vi "ConfigureCameraImage.vi"(10 "Image Type":T3 items=["Grayscale (U8)", "Grayscale (I16)", "Grayscale (SGL)", "Complex (CSG)", "RGB (U32)", "HSL (U32)", "RGB (U64)", "Grayscale (U16)"], 11 "Refnum in":T1="cam0") -> (1 "Camera Image":T2, 3 "Refnum out":T1)   [LabVIEW 2013]
doc: "Configure the stuff needed to talk to the camera above the pool for the little boats."
uses:
  <vilib>/userdefined/High Color/IMAQdx.ctl
  <vilib>/vision/Image Controls.llb/IMAQ Image.ctl
  <vilib>/vision/driver/NI_Vision_Acquisition_Software.lvlib
panel:
  out "error out":errorcluster
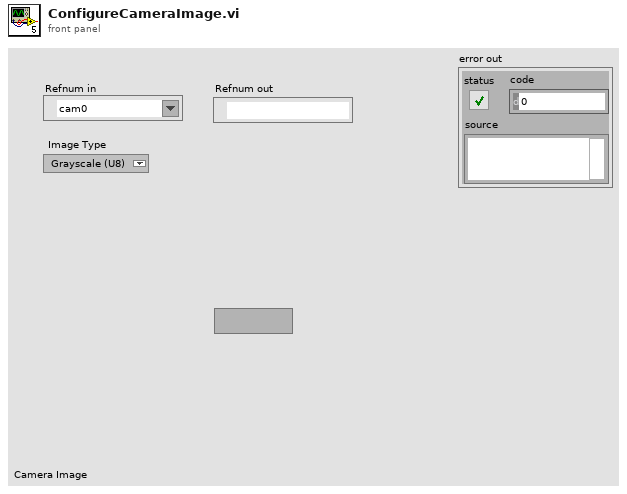
[diagram p1: front panel]
types:
  T1 = typedef "IMAQdx.ctl" = refnum<k21>
  T2 = typedef "IMAQ Image.ctl" = refnum<image>
  T3 = typedef "Image Type" = u32
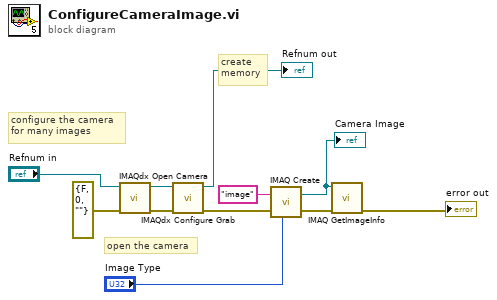
[diagram p0: block diagram]
diagram:
  # "create\nmemory"
  # "configure the camera\nfor many images"
  # "open the camera"
  n1 = call <vilib>:"IMAQdx Open Camera.vi"("error in"=errorcluster {"status"=FALSE, "code"=0, "source"=""}, "Session In"="Refnum in") -> ("error out"=w5:errorcluster, "Session Out"=w4:T1)  [unwired: 1 in, 7 out]
  n2 = call <vilib>:"IMAQdx Configure Grab.vi"("error in"=w5, "Session In"=w4) -> ("error out"=w3:errorcluster, "Session Out"=→"Refnum out":T1)  [unwired: 8 out]
  n3 = call "IMAQ Create"("Image Name"="image", "Image Type"="Image Type", "error in (no error)"=w3) -> ("New Image"=w9:T2, "error out"=w2:errorcluster)  [unwired: 1 in, 1 out]
  "Camera Image" <- w9
  n4 = call "IMAQ GetImageInfo"("error in (no error)"=w2, "Image"=w9) -> ("error out"=→"error out":errorcluster)  [unwired: 2 in, 7 out]
